vi "Step Status.vi"(6 "Status Notifier":refnum<notifier>, 8 "Start Time":dbl, 9 "Action":i32, 10 "Run":i32, 11 "Maze":i32) -> (3 "Timeout?":bool)   [LabVIEW 2020]
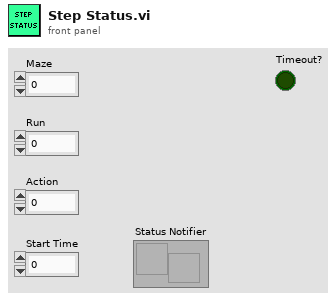
[diagram p1: front panel]
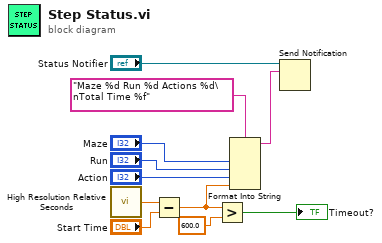
[diagram p0: block diagram]
diagram:
  n1 = call <vilib>:"High Resolution Relative Seconds.vi"() -> ("relative seconds"=w10:dbl)
  n2 = Subtract(x=w10, y="Start Time") -> (x-y=w3:dbl)
  n3 = Greater?(x=w3, y=600.0) -> (0:→"Timeout?":bool)
  n4 = Format Into String(format string="Maze %d Run %d Actions %d\nTotal Time %f", "Maze", "Run", "Action", w3) -> (resulting string=w1:string)  [unwired: 2 in, 1 out]
  n5 = Send Notification(notification=w1, notifier="Status Notifier") -> ()  [unwired: 1 in, 2 out]
